vi "Format DateTime String.vi"(11 "time stamp":timestamp) -> (3 "date/time string":string)   [LabVIEW 2011]
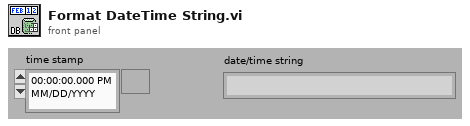
[diagram p1: front panel]
types:
  T1 = typedef "LVDateTimeRec.ctl" = cluster{"fractional second":dbl, "second":i32, "minute":i32, "hour":i32, "day of month":i32, "month":i32, "year":i32, "day of week":i32, "day of year":i32, "DST":i32}
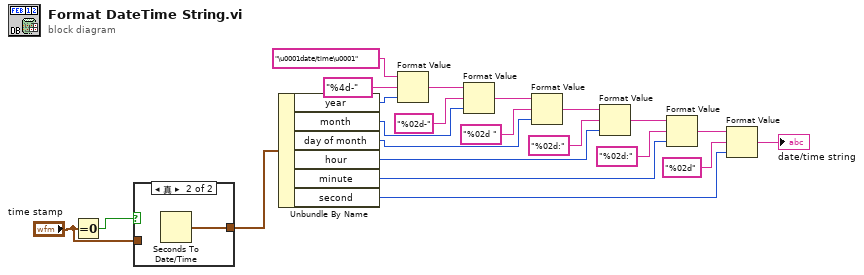
[diagram p0: block diagram]
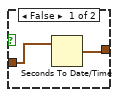
[diagram p2: hidden frame]
diagram:
  n1 = Equal To 0?(x="time stamp") -> (x = 0?=w21:bool)
  n2 = case shown="真" w21 {
    tunnel: [w23 w25] -> w20
    tunnel: "time stamp" -> [w24 _]
    frame False {
      n3 = Seconds To Date/Time(time stamp (now)=w24) -> (date time rec=w23:T1)  [unwired: 1 in]
    }
    frame True {
      n4 = Seconds To Date/Time() -> (date time rec=w25:T1)  [unwired: 2 in]
    }
  }
  n5 = Unbundle By Name(w20) -> ("year"=w13:i32, "month"=w14:i32, "day of month"=w15:i32, "hour"=w1:i32, "minute"=w4:i32, "second"=w5:i32)
  n6 = Format Value(string ("")="\u0001date/time\u0001", format string="%4d-", value (0)=w13) -> (output string=w10:string)
  n7 = Format Value(string ("")=w10, format string="%02d-", value (0)=w14) -> (output string=w11:string)
  n8 = Format Value(string ("")=w11, format string="%02d ", value (0)=w15) -> (output string=w12:string)
  n9 = Format Value(string ("")=w12, format string="%02d:", value (0)=w1) -> (output string=w2:string)
  n10 = Format Value(string ("")=w2, format string="%02d:", value (0)=w4) -> (output string=w3:string)
  n11 = Format Value(string ("")=w3, format string="%02d", value (0)=w5) -> (output string=→"date/time string":string)
